vi "Result_Test.vi"(8 "error in (no error)":errorcluster caption="entrée d'erreur (pas d'erreur)", 11 "Nodon_Get_BP_Status IN":refnum<class "Nodon_Get_Switch_Status.lvclass">) -> (0 "error out":errorcluster caption="sortie d'erreur", 3 "Nodon_Get_BP_Status OUT":refnum<class "Nodon_Get_Switch_Status.lvclass">)   [LabVIEW 2020, in "Library Test.lvlib" / "Nodon_Get_Switch_Status.lvclass"]
uses:
  Nodon_Get_Switch_Status.lvclass
  C:/Users/ngarcin/OneDrive - Altyor/Standard TB/Suite TB45/Class/Test/Test (Default)/Test (Default).lvclass
  Commun VI/TypeDef/Variable Printable.ctl
  JSON API/JSON Value/Set from JSON string.vi
  JSON API/JSON Value/JSON Value.lvclass
  Nodon_Send_Command_UART/Nodon_Send_Command_UART.lvclass
  JSON API/Variant JSON/Variant JSON.lvlib
  JSON API/Get Polymorphic/JSON GetSet.lvlib
  Commun VI/Library Commun.lvlib
panel:
  out "données":string
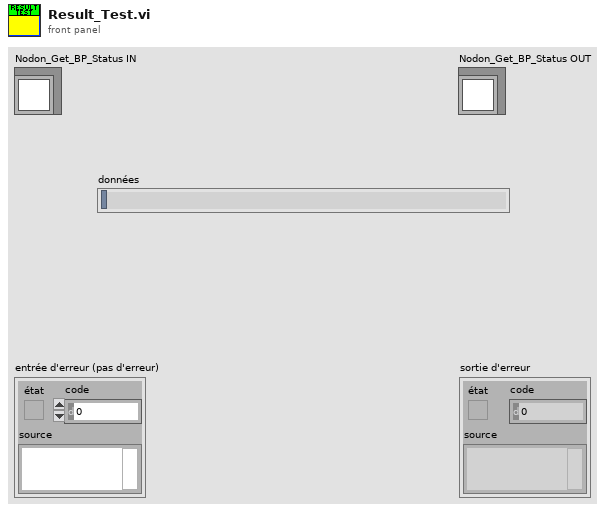
[diagram p1: front panel]
types:
  T1 = typedef "Variable Printable.ctl" = string
  T2 = enum16{"Get Variable", "Get All Variables", "Set Variable", "Delete Variable", "Delete All Variable"}
  T3 = cluster{"Commande Type":string, "Command ID":string, "Data":string, "Error":string}
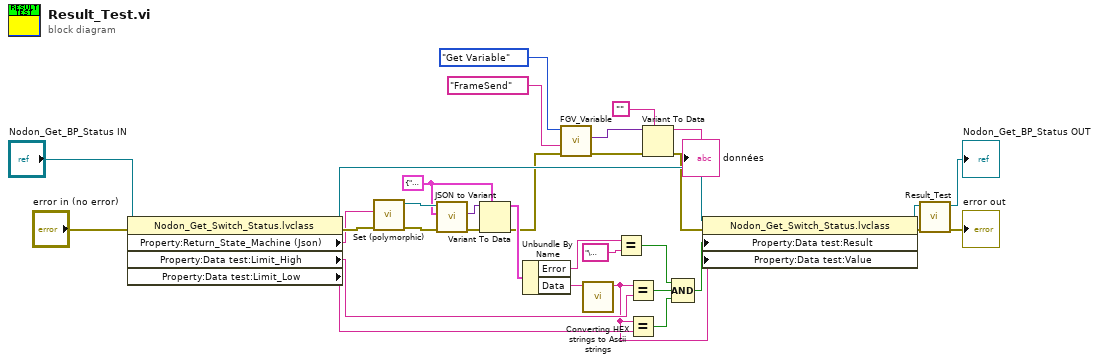
[diagram p0: block diagram]
diagram:
  w21 = T3 {"Commande Type"="", "Command ID"="", "Data"="", "Error"=""}
  n1 = property class="Nodon_Get_Switch_Status.lvclass"(reference="Nodon_Get_BP_Status IN", error in="error in (no error)") -> (reference out=w31:refnum<class "Nodon_Get_Switch_Status.lvclass">, error out=w26:errorcluster, "Property:Return_State_Machine (Json)"=w25:string, "Property:Data test:Limit_High"=w14:string, "Property:Data test:Limit_Low"=w13:string)
  n2 = call-poly "Set (polymorphic).vi"("error in (no error)"=w26, "JSON stream"=w25) -> ("error out"=w28:errorcluster, "JSON Value out"=w30:refnum<class "JSON Value.lvclass">)  [unwired: 7 in, 1 out]
  n3 = call "JSON to Variant.vi"("error in (no error)"=w28, "Variant (Data Type)"=w21, "JSON Value"=w30) -> ("error out"=w29:errorcluster, "Variant out"=w27:variant)  [unwired: 7 in]
  n4 = Variant To Data(error in=w29, type=w21, Variant=w27) -> (data=w24:T3, error out=w3:errorcluster)
  n5 = Unbundle By Name(w24) -> ("Error"=w23:string, "Data"=w16:string)
  n6 = call "FGV_Variable.vi"("error in (no error)"=w3, "Variable"=T1 "FrameSend", "Function"=T2."Get Variable") -> ("error out"=w4:errorcluster, "Data Out"=w5:variant)  [unwired: 6 in, 1 out]
  n7 = call "Converting HEX strings to Ascii strings.vi"("chaîne IN"=w16) -> ("Chaîne OUT"=w12:string)  [unwired: 9 in, 1 out]
  n8 = Equal?(x=w23, y="\u0000") -> (x = y?=w10:bool)
  n9 = Equal?(x=w12, y=w14) -> (x = y?=w15:bool)
  n10 = Equal?(x=w12, y=w13) -> (x = y?=w11:bool)
  n11 = Variant To Data(error in=w4, type="", Variant=w5) -> (data=→"données":string, error out=w2:errorcluster)
  n12 = Compound Arithmetic op=AND ("Opérateur arithmétique")(w10, w15, w11) -> (w9:bool)
  n13 = property class="Nodon_Get_Switch_Status.lvclass"(reference=w31, error in=w2, "Property:Data test:Result"=w9, "Property:Data test:Value"=w12) -> (reference out=w18:refnum<class "Nodon_Get_Switch_Status.lvclass">, error out=w17:errorcluster)
  n14 = call-parent "Result_Test.vi"("error in (no error)"=w17, "Get_Voltage en entrée"=w18) -> ("error out"=→"error out":errorcluster, "Get_Voltage en sortie"=→"Nodon_Get_BP_Status OUT":refnum<class "Nodon_Get_Switch_Status.lvclass">)  [unwired: 8 in]
